vi "Set Column Header.vi"(8 "error in (no error)":errorcluster, 9 "Column Index":i32, 10 "Column Name":string, 11 "Main Display in":refnum<class "Main Display.lvclass">) -> (0 "error out":errorcluster, 3 "Main Display out":refnum<class "Main Display.lvclass">)   [LabVIEW 2016, in "Assert API Components.lvlib" / "Assert Display.lvlib" / "Main Display.lvlib" / "Main Display.lvclass"]
uses:
  Main Display.lvclass
  Main Display.lvclass/Main Display.ctl
  Display Configurations/Base Display Configuration.lvclass/Base Display Configuration.ctl
  Display Configurations/Base Display Configuration.lvclass
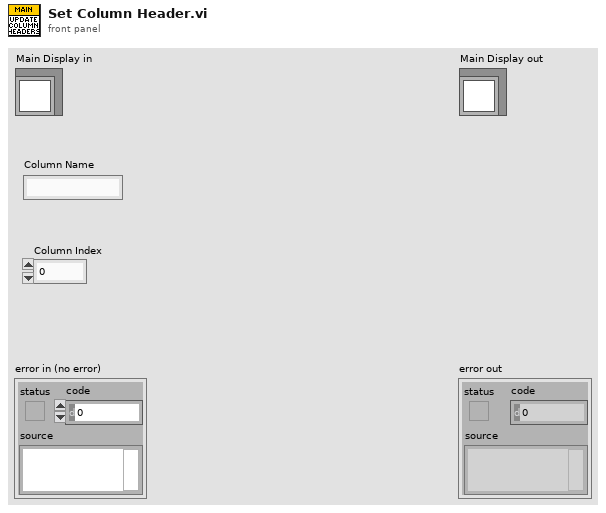
[diagram p1: front panel]
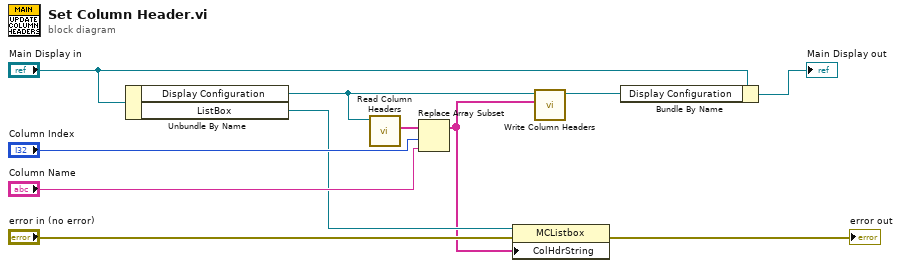
[diagram p0: block diagram]
diagram:
  n1 = Unbundle By Name("Main Display in") -> ("Display Configuration"=w9:refnum<class "Base Display Configuration.lvclass">, "ListBox"=w6:refnum<vi>)
  n2 = call "Read Column Headers.vi"("Base Display Configuration in"=w9) -> ("Column Headers"=w10:string[])  [unwired: 10 in]
  n3 = Replace Array Subset(array=w10, new element="Column Name", index="Column Index") -> (w4:string[])
  n4 = property class="MCListbox"(reference=w6, error in="error in (no error)", "ColHdrString"=w4) -> (error out=→"error out":errorcluster)  [unwired: 1 out]
  n5 = call "Write Column Headers.vi"("Column Headers"=w4, "Base Display Configuration in"=w9) -> ("Base Display Configuration out"=w1:refnum<class "Base Display Configuration.lvclass">)  [unwired: 9 in]
  n6 = Bundle By Name(cluster="Main Display in", "Display Configuration"=w1) -> (→"Main Display out":refnum<class "Main Display.lvclass">)
